vi "NetComm_getJoystickButtons.vi"(8 "error in (no error)":errorcluster, 11 "Joystick Number":i32) -> (0 "error out":errorcluster, 2 "Buttons":bool[](array[boolean]))   [LabVIEW 2017]
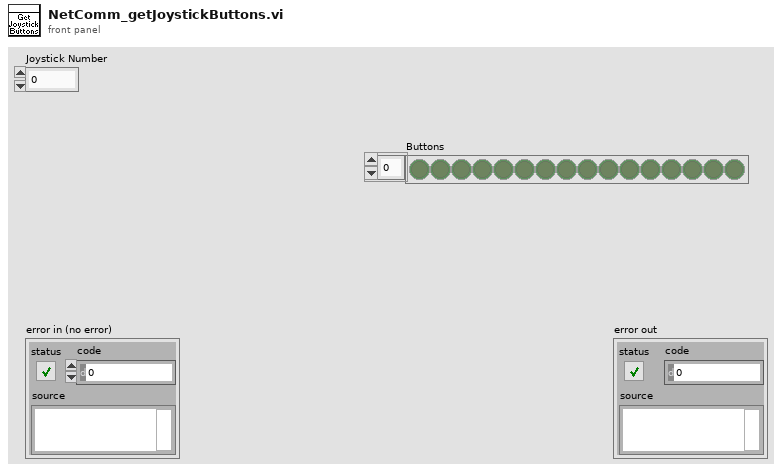
[diagram p1: front panel]
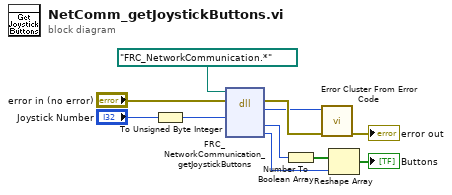
[diagram p0: block diagram]
diagram:
  n1 = To Unsigned Byte Integer(number="Joystick Number") -> (unsigned 8bit integer=w6:u8)
  n2 = dll-call lib="?" fn="FRC_NetworkCommunication_getJoystickButtons"(path in=path "FRC_NetworkCommunication.*", error in="error in (no error)", "joystickNum"=w6) -> (error out=w8:errorcluster, "return type"=w7:i32, "buttons"=w3:u32, "count"=w5:u8)  [unwired: 4 in, 1 out]
  n3 = Number To Boolean Array(number=w3) -> (Boolean array=w2:bool[])
  n4 = call <vilib>:"Error Cluster From Error Code.vi"("error in (no error)"=w8, "error code (0)"=w7) -> ("error out"=→"error out":errorcluster)  [unwired: 7 in]
  n5 = Reshape Array(w2, w5) -> (→"Buttons":bool[])
